vi "Save to File.vi"(0 "Neural Network In":T1={"Weigths"=[], "Last Layer Linear"=TRUE, "Add Bias Inputs"=TRUE, "# Inputs"=0, "# Output Neurons/Outputs"=0, "Inputs Scaling"={"X Scaling Vector"=[], "Y Scaling Vector"=[]}, "Outputs Scaling"={"X Scaling Vector"=[], "Y Scaling Vector"=[]}}, 5 "File Path (dialog)":path, 11 "Error In":errorcluster) -> (6 "Path Used":path, 10 "Cancelled":bool, 15 "Error Out":errorcluster)   [LabVIEW 2013, in "Super Simple Neural Network.lvlib"]
doc: "This VI saves the neural network to a file."
uses:
  Super Simple Neural Network.lvlib
  Types/Neural Network.ctl
  Types/2D Array.ctl
  Types/Scaling Info.ctl
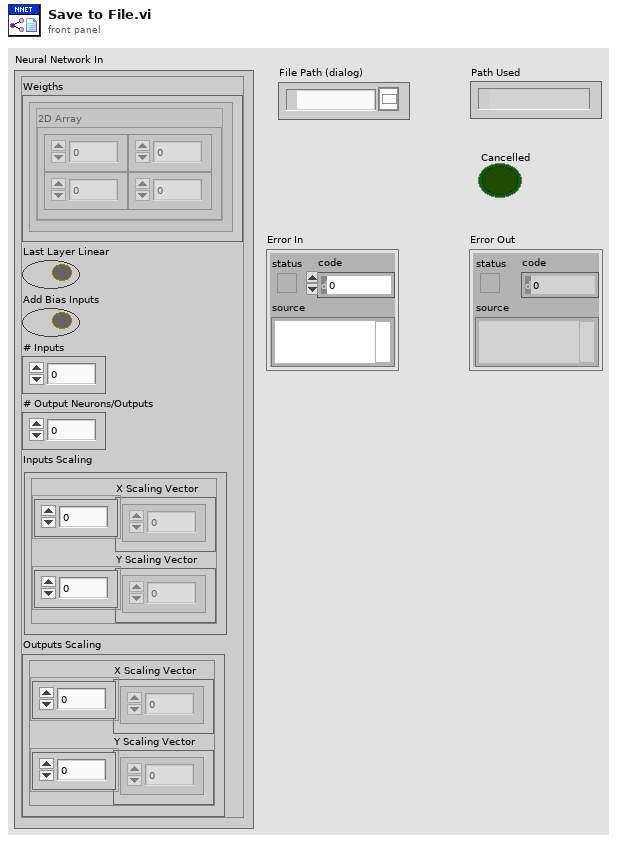
[diagram p1: front panel]
types:
  T1 = typedef "Super Simple Neural Network.lvlib/Neural Network.ctl" = cluster{"Weigths":T2[], "Last Layer Linear":bool, "Add Bias Inputs":bool, "# Inputs":u32, "# Output Neurons/Outputs":u32, "Inputs Scaling":T3, "Outputs Scaling":T3}
  T2 = typedef "Super Simple Neural Network.lvlib/2D Array.ctl" = cluster{"2D Array":dbl[][]}
  T3 = typedef "Super Simple Neural Network.lvlib/Scaling Info.ctl" = cluster{"X Scaling Vector":dbl[], "Y Scaling Vector":dbl[]}
  T4 = enum16{"open", "replace", "create", "open or create", "replace or create", "replace or create with confirmation"}
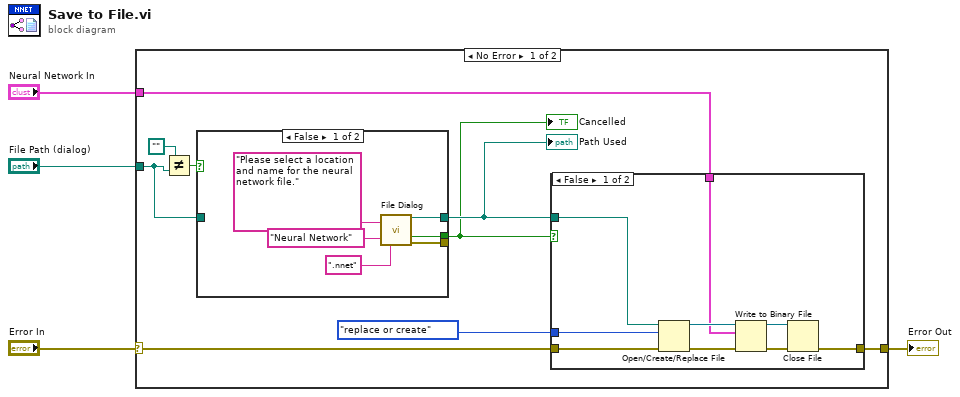
[diagram p0: block diagram]
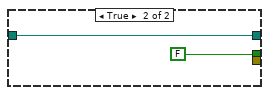
[diagram p3: hidden frame]
diagram:
  n1 = case shown="No Error" "Error In" {
    selector: "Error In" -> [w12 w32]
    tunnel: [w10 w32] -> w3
    tunnel: "Neural Network In" -> [w11 _]
    tunnel: "File Path (dialog)" -> [w6 _]
    frame No Error {
      n2 = Not Equal?(x=path "", y=w6) -> (x != y?=w7:bool)
      n3 = case shown="False" w7 {
        tunnel: [w26 w31] -> w13
        tunnel: w6 -> [_ w31]
        tunnel: [w25 FALSE ("cancelled")] -> w9
        tunnel: [w24 _] -> _
        frame False {
          n4 = call "File Dialog"("prompt"="Please select a location and name for the neural network file.", "pattern (all files)"=".nnet", "pattern label"="Neural Network") -> ("selected path"=w26:path, "cancelled"=w25:bool, "error out"=w24:errorcluster)  [unwired: 9 in, 1 out]
        }
        frame True {
        }
      }
      "Cancelled" <- w9
      "Path Used" <- w13
      n5 = case shown="False" w9 {
        tunnel: w13 -> [w22 _]
        tunnel: w12 -> [w20 w23]
        tunnel: w11 -> [w18 _]
        tunnel: [w15 w23] -> w10
        tunnel: T4."replace or create" ("operation (0:open)") -> [w14 _]
        frame False {
          n6 = Open/Create/Replace File(file path (use dialog)=w22, error in=w20, operation (0:open)=w14) -> (refnum out=w21:refnum<file>, error out=w19:errorcluster)  [unwired: 3 in, 1 out]
          n7 = Write to Binary File(file (use dialog)=w21, data=w18, error in=w19) -> (refnum out=w17:refnum<file>, error out=w16:errorcluster)  [unwired: 3 in, 1 out]
          n8 = Close File(refnum=w17, error in=w16) -> (error out=w15:errorcluster)  [unwired: 1 out]
        }
        frame True {
        }
      }
    }
    frame Error {
    }
  }
  "Error Out" <- w3
